vi "Extract HW Config.vi"(9 "Ring Refnum":refnum<vi>, 11 "Configuration Folder Path":path) -> (3 "Channel 2":T1[](array[typedef]) {"Stop Bit" items=["1.0", "1.5", "2.0"]; "Parity" items=["None", "Odd", "Even", "Mark", "Space"]})   [LabVIEW 2020]
uses:
  Port details.ctl
panel:
  in  "Channel 1":T1[](array[typedef]) {"Stop Bit" items=["1.0", "1.5", "2.0"]; "Parity" items=["None", "Odd", "Even", "Mark", "Space"]}
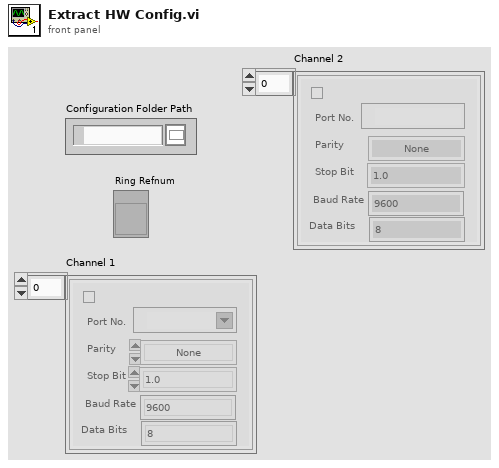
[diagram p1: front panel]
types:
  T1 = typedef "Port details.ctl" = cluster{"Port No.":refnum<visa-resource-name>, "Checkbox":bool, "Parity":u16, "Stop Bit":u16, "Baud Rate":u32, "Data Bits":u8}
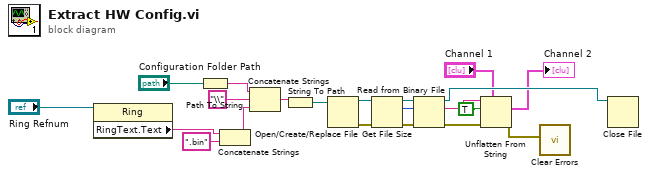
[diagram p0: block diagram]
diagram:
  n1 = property on="Property Node" class="Ring"(reference="Ring Refnum") -> ("RingText.Text"=w14:string)  [unwired: 1 in, 2 out]
  n2 = Path To String(path="Configuration Folder Path") -> (string=w11:string)
  n3 = Concatenate Strings(w14, ".bin" ("string")) -> (w16:string)
  n4 = Concatenate Strings(w11, "\\" ("string"), w16) -> (w13:string)
  n5 = String To Path(string=w13) -> (path=w10:path)
  n6 = Open/Create/Replace File(file path (use dialog)=w10) -> (refnum out=w21:refnum<file>, error out=w20:errorcluster)  [unwired: 5 in, 1 out]
  n7 = Get File Size(file=w21, error in=w20) -> (refnum out=w18:refnum<file>, size (in bytes)=w4:i64, 0:w19:errorcluster)
  n8 = Read from Binary File(8:w19, 10:w4, 11:w18) -> (0:w6:errorcluster, 2:w9:string, 3:w17:refnum<file>)  [unwired: 3 in, 1 out]
  n9 = Unflatten From String(type="Channel 1", binary string=w9, data includes array or string size? (T)=TRUE, error in (no error)=w6) -> (value=→"Channel 2":T1[], error out=w5:errorcluster)  [unwired: 1 in, 1 out]
  n10 = call <vilib>:"Clear Errors.vi"("error in (no error)"=w5) -> ()  [unwired: 5 in, 2 out]
  n11 = Close File(refnum=w17) -> ()  [unwired: 1 in, 2 out]
